vi "configure.vi"(8 "error in (no error)":errorcluster, 11 "DL090324Microscope in":refnum<class "InstrumentDL090324.lvclass">) -> (0 "error out":errorcluster, 3 "DL090324Microscope out":refnum<class "InstrumentDL090324.lvclass">)   [LabVIEW 2010, in "InstrumentDL090324.lvclass"]
uses:
  InstrumentDL090324.lvclass
  common/classes/GenericComponent/GenericComponent/GenericComponent.lvclass
  Detector/GenericDetector/GenericDetector/GenericDetector.lvclass
  LightSource/GenericLightSource/GenericLightSource/GenericLightSource.lvclass
panel:
  out "LSID":string
  in  "Tab Control":T1(tab)
  in  "configure detectors":bool
  in  "configure light source":bool
  out "Configuration":string
  in  "cancel button":bool
  in  "save button":bool
  # "Configure InstrumentDL090324"
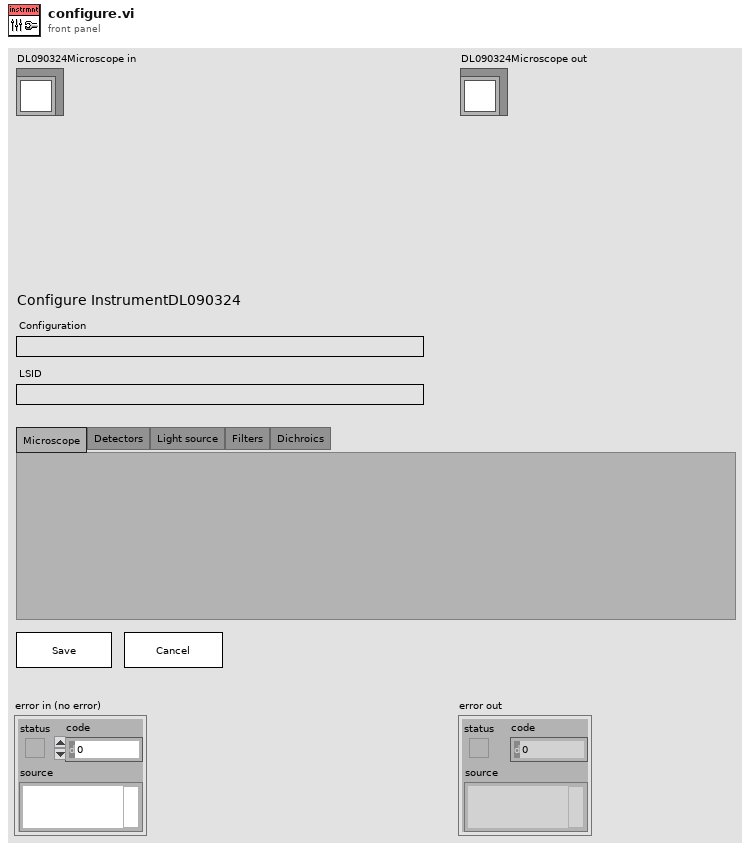
[diagram p1: front panel]
types:
  T1 = enum32{"Microscope", "Detectors", "Light source", "Filters", "Dichroics"}
  T2 = typedef "LSID_cluster.ctl" = cluster{"identifier":string, "revision":i32}
  T3 = typedef "plugin_specification.ctl" = cluster{"class path":string, "configuration":string, "label":string, "settings name":string}
  T4 = typedef "InstrumentDL090324.lvclass/config_data_cluster.ctl" = cluster{"detectors":T3[], "LSID":T2, "light source":T3[]}
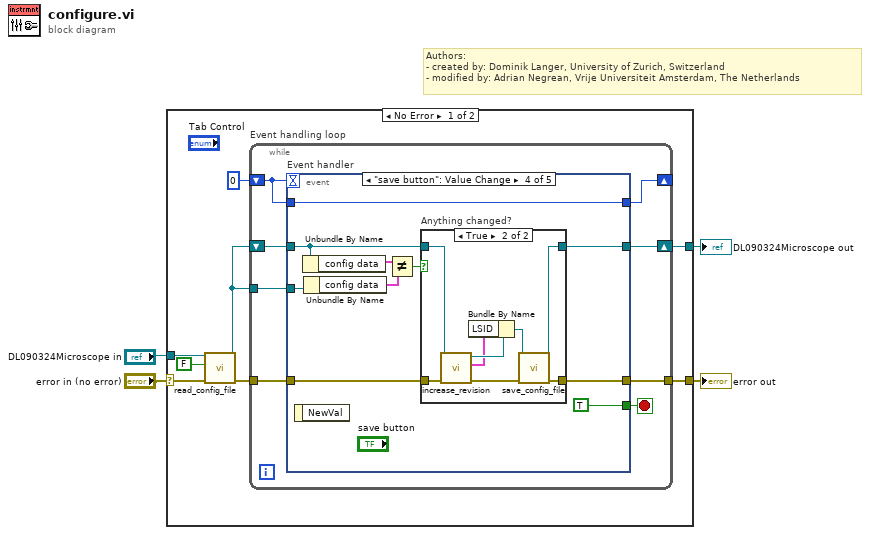
[diagram p0: block diagram]
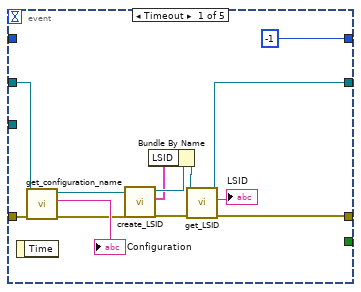
[diagram p2: hidden frame]
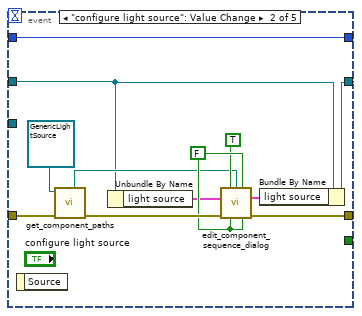
[diagram p3: hidden frame]
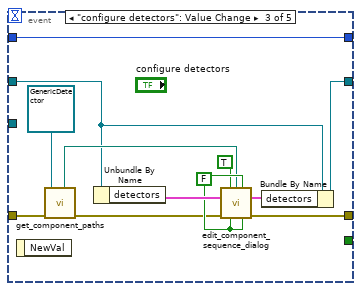
[diagram p4: hidden frame]
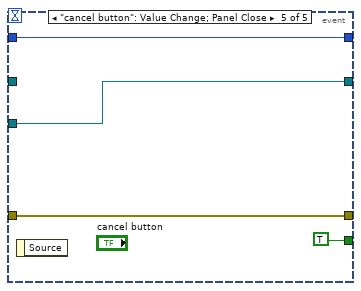
[diagram p6: hidden frame]
diagram:
  # "Authors: \n- created by: Dominik Langer, University of Zurich, Switzerland\n- modified by: Adrian Negrean, Vrije Universiteit Amsterdam, The Netherlands"
  n1 = case shown="No Error" "error in (no error)" {
    selector: "error in (no error)" -> [w10 w82]
    tunnel: [w12 w82] -> w3
    tunnel: [w6 w81] -> w1
    tunnel: "DL090324Microscope in" -> [w7 w81]
    frame No Error {
      n2 = call-dynamic "read_config_file.vi"("error in (no error)"=w10, "force load?"=FALSE, "GenericPlugin in"=w7) -> ("error out"=w9:errorcluster, "GenericPlugin out"=w5:refnum<class "InstrumentDL090324.lvclass">)  [unwired: 7 out]
      n3 = while "Event handling loop" {
        tunnel: w9 -> [w20]
        tunnel: [w19] -> w12
        shift-right: [w17] -> _
        shift-left: 0 -> [w18]
        shift-right: [w15] -> w6
        shift-left: w5 -> [w16]
        tunnel: w5 -> [w13]
        stop <- w14 stop-if-true
        n4 = event "Event handler" shown="[3] \"save button\": Value Change" {
          selector: _ -> [_ _ _ _ _]
          dyn-events: _ -> [_ _ _ _ _]
          timeout: w18 -> [_ _ _ _ _]
          tunnel: w20 -> [w31 w44 w49 w64 w80]
          tunnel: [w21 w44 w55 w58 w80] -> w19
          tunnel: w18 -> [_ w43 w56 w66 w79]
          tunnel: [-1 w43 w56 w66 w79] -> w17
          tunnel: [w26 w36 w52 w57 w77] -> w15
          tunnel: w16 -> [w30 w37 w45 w63 _]
          tunnel: [_ _ _ TRUE TRUE] -> w14
          tunnel: w13 -> [_ _ _ w60 w77]
          event Timeout {
            n5 = event-data() -> ()  [unwired: 2 out]
            n6 = call "get_configuration_name.vi"("error in (no error)"=w31, "GenericPlugin.lvclass in"=w30) -> ("error out"=w22:errorcluster, "configuration name"=→"Configuration":string, "GenericPlugin.lvclass out"=w27:refnum<class "InstrumentDL090324.lvclass">)  [unwired: 7 in]
            n7 = call-dynamic "create_LSID.vi"("error in (no error)"=w22, "GenericPlugin in"=w27) -> ("error out"=w28:errorcluster, "current LSID"=w23:T2, "GenericPlugin out"=w25:refnum<class "InstrumentDL090324.lvclass">)  [unwired: 7 in]
            n8 = Bundle By Name(cluster=w25, "LSID"=w23) -> (w24:refnum<class "InstrumentDL090324.lvclass">)
            n9 = call-dynamic "get_LSID.vi"("error in (no error)"=w28, "GenericPlugin in"=w24) -> ("error out"=w21:errorcluster, "LSID (string)"=→"LSID":string, "GenericPlugin out"=w26:refnum<class "InstrumentDL090324.lvclass">)  [unwired: 6 in, 1 out]
          }
          event "configure light source": Value Change {
            w41 = FALSE ("show label?")
            n10 = event-data() -> ()  [unwired: 2 out]
            n11 = call-dynamic "get_component_paths.vi"("GenericComponent in"=refnum<class "GenericLightSource.lvclass"> refnum ("GenericLightSource.lvclass")) -> ("error out"=w39:errorcluster, "component type directory"=w38:path)  [unwired: 5 in, 4 out]
            n12 = Unbundle By Name(w37) -> ("light source"=w35:T3[])
            n13 = call "edit_component_sequence_dialog.vi"("show configuration?"=TRUE, "default folder path"=w38, "show label?"=w41, "component specification list in"=w35, "error in (no error)"=w39, "choose default?"=w41, "show settings?"=w41) -> ("component specification list out"=w42:T3[])  [unwired: 6 in, 2 out]
            n14 = Bundle By Name(cluster=w37, "light source"=w42) -> (w36:refnum<class "InstrumentDL090324.lvclass">)
          }
          event "configure detectors": Value Change {
            w51 = FALSE ("show label?")
            n15 = event-data() -> ()  [unwired: 2 out]
            n16 = call-dynamic "get_component_paths.vi"("error in (no error)"=w49, "GenericComponent in"=refnum<class "GenericDetector.lvclass"> refnum ("GenericDetector.lvclass")) -> ("error out"=w48:errorcluster, "component type directory"=w46:path)  [unwired: 4 in, 4 out]
            n17 = Unbundle By Name(w45) -> ("detectors"=w54:T3[])
            n18 = call "edit_component_sequence_dialog.vi"("show configuration?"=TRUE, "default folder path"=w46, "show label?"=w51, "component specification list in"=w54, "error in (no error)"=w48, "choose default?"=w51, "show settings?"=w51) -> ("component specification list out"=w53:T3[], "error out"=w55:errorcluster)  [unwired: 6 in, 1 out]
            n19 = Bundle By Name(cluster=w45, "detectors"=w53) -> (w52:refnum<class "InstrumentDL090324.lvclass">)
          }
          event "save button": Value Change {
            n20 = event-data() -> ()  [unwired: 2 out]
            n21 = Unbundle By Name(w63) -> ("config data"=w61:T4)
            n22 = Unbundle By Name(w60) -> ("config data"=w59:T4)
            n23 = Not Equal?(x=w61, y=w59) -> (x != y?=w62:bool)
            n24 = case "Anything changed?" shown="True" w62 {
              tunnel: w64 -> [w68 w76]
              tunnel: [w68 w70] -> w58
              tunnel: w63 -> [w67 w73]
              tunnel: [w67 w69] -> w57
              frame False {
              }
              frame True {
                n25 = call-dynamic "increase_revision.vi"("error in (no error)"=w76, "GenericPlugin in"=w73) -> ("error out"=w71:errorcluster, "new LSID"=w74:T2, "GenericPlugin out"=w75:refnum<class "InstrumentDL090324.lvclass">)  [unwired: 7 in]
                n26 = Bundle By Name(cluster=w75, "LSID"=w74) -> (w72:refnum<class "InstrumentDL090324.lvclass">)
                n27 = call-dynamic "save_config_file.vi"("error in (no error)"=w71, "GenericPlugin in"=w72) -> ("error out"=w70:errorcluster, "GenericPlugin out"=w69:refnum<class "InstrumentDL090324.lvclass">)  [unwired: 1 in, 7 out]
              }
            }
          }
          event "cancel button": Value Change; Panel Close {
            n28 = event-data() -> ()  [unwired: 2 out]
          }
        }
      }
    }
    frame Error {
    }
  }
  "error out" <- w3
  "DL090324Microscope out" <- w1
